vi "Main.vi"(0 "Door open":bool, 5 "Stop":bool, 7 "Start":bool, 9 "Cancel":bool, 11 "Error in":errorcluster) -> (4 "Recipe":i32(listbox), 6 "Cooking":bool, 8 "Power Level":i32, 10 "Buzzer":bool, 14 "Display Panel":string, 15 "Error out":errorcluster)   [LabVIEW 2020, in "Microwave oven.lvlib"]
doc: "This machine is the implementation of microwave oven which will get available food items from a csv file and cook it and display the power level in the front panel indicator"
uses:
  Microwave oven.lvlib
  Typedefs/Queue driver operations.ctl
  Typedefs/Data cluster.ctl
  Typedefs/Number values.ctl
  Typedefs/Timer details.ctl
panel:
  in  "Nine 9":bool
  in  "Eight 8":bool
  in  "Seven 7":bool
  in  "Six 6":bool
  in  "Five 5":bool
  in  "Four 4":bool
  in  "Three 3":bool
  in  "Two 2":bool
  in  "One 1":bool
  # "MICROWAVE OVEN"
  # "MICROWAVE OVEN"
  # "INSTRUCTIONS:\n1. The available recipes are displayed\nin recipes.\n2. You can select the required recipe\nfrom keypad.\n3. Click start to start cooking.\n4. You cannot open the door during\nthe cooking process .\n5. You cannot select another food to \ncook during the cooking process"
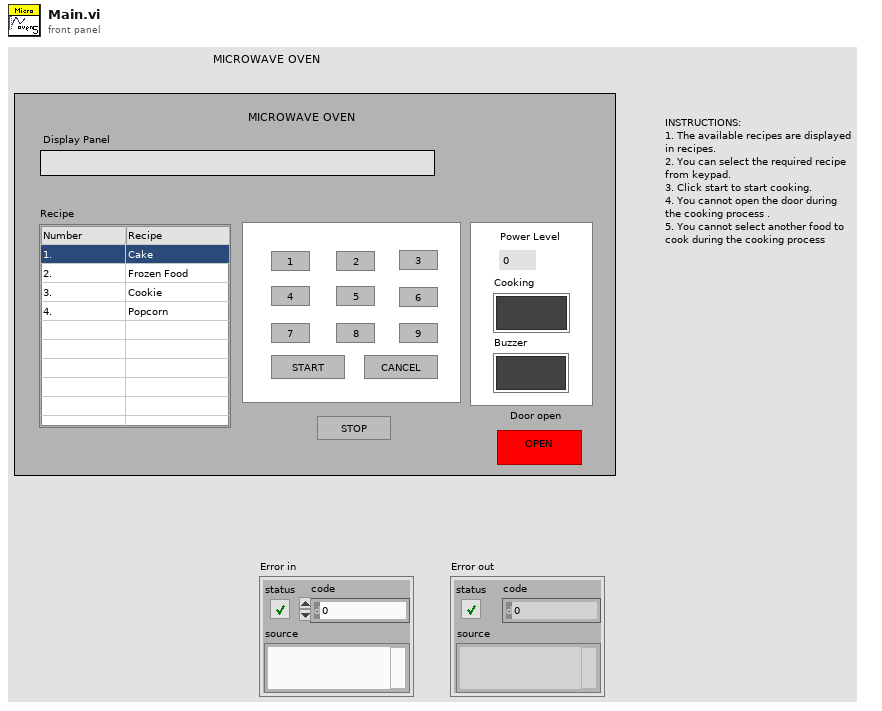
[diagram p1: front panel]
types:
  T1 = typedef "Microwave oven.lvlib/Data cluster.ctl" = cluster{"Number":T2, "Start":bool, "Stop":bool, "Cancel":bool, "Door open":bool, "Power Level":i32, "Display Panel":string, "Cooking":bool, "Buzzer":bool, "Timer details":T3, "Enable controls ref":refnum<vi>[], "Disable controls ref":refnum<vi>[], "Path":path, "Recipe":i32, "Recipie index":i32, "Current Step":i32, "Total Steps":i32, "Recipe Name":string, "Full Recipe":string[], "Recipe Book":string[][], "Cooking time":i32, "Boolean ref":refnum<vi>[]}
  T2 = typedef "Microwave oven.lvlib/Number values.ctl" = cluster{"One":bool, "Two":bool, "Three":bool, "Four":bool, "Five":bool, "Six":bool, "Seven":bool, "Eight":bool, "Nine":bool}
  T3 = typedef "Microwave oven.lvlib/Timer details.ctl" = cluster{"Started?":bool, "Paused":bool, "Start time":dbl, "Set time":dbl, "Previous time":dbl, "Elapsed time":dbl}
  T4 = typedef "Microwave oven.lvlib/Queue driver operations.ctl" = enum16{"Create queue", "Enqueue", "Enstack", "Dequeue", "Flush", "Release"}
  T5 = enum16{"open", "replace", "create", "open or create", "replace or create", "replace or create with confirmation"}
  T6 = enum8{"Enabled", "Disabled", "Disabled and Grayed Out"}
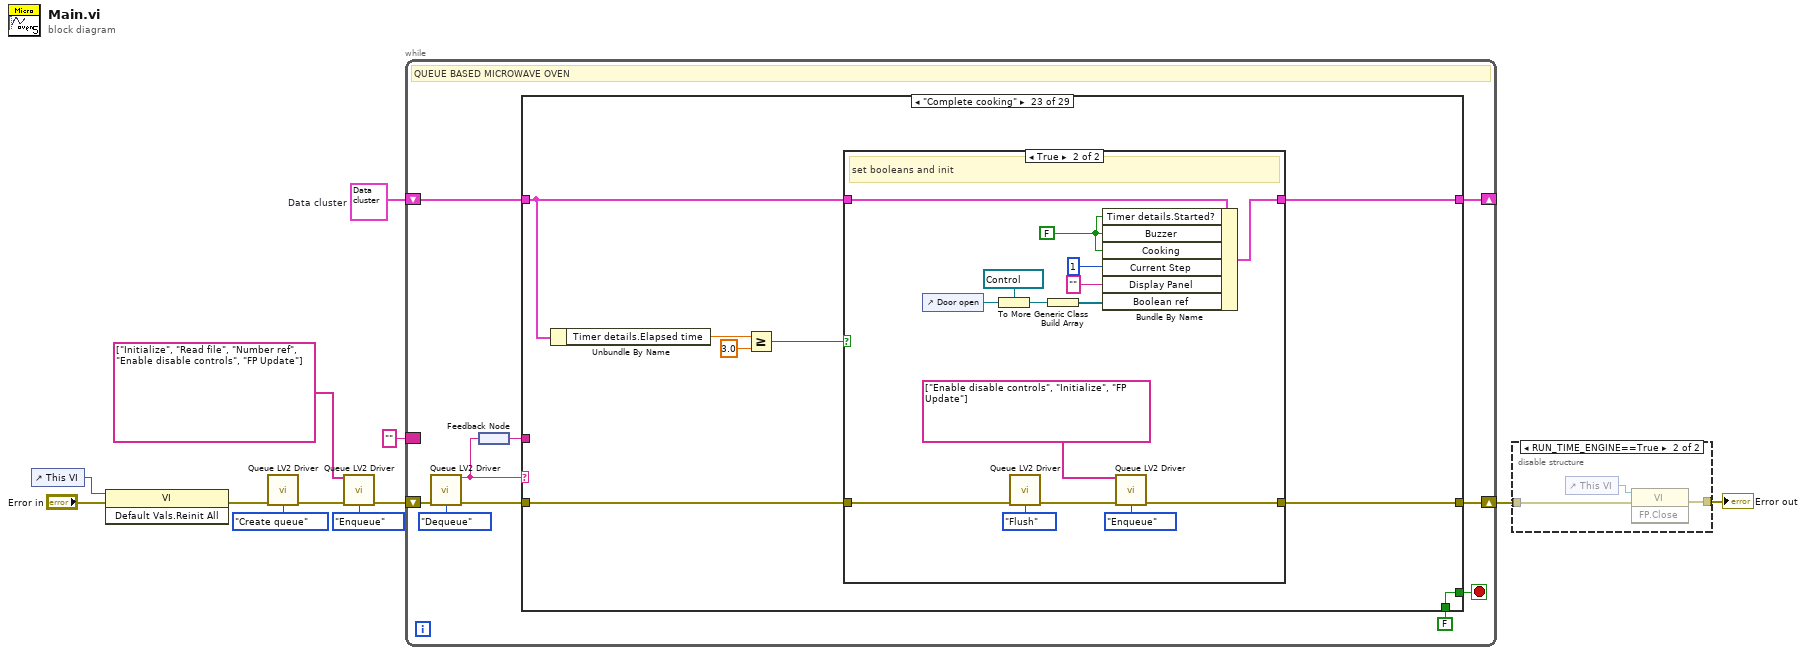
[diagram p0: block diagram]
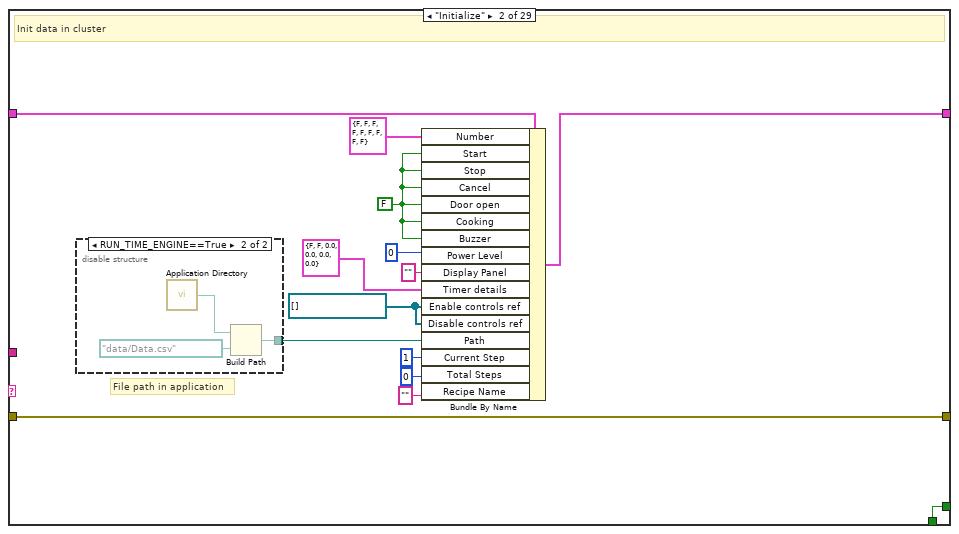
[diagram p4: hidden frame]
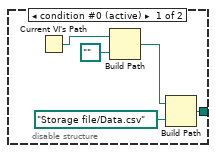
[diagram p5: hidden frame]
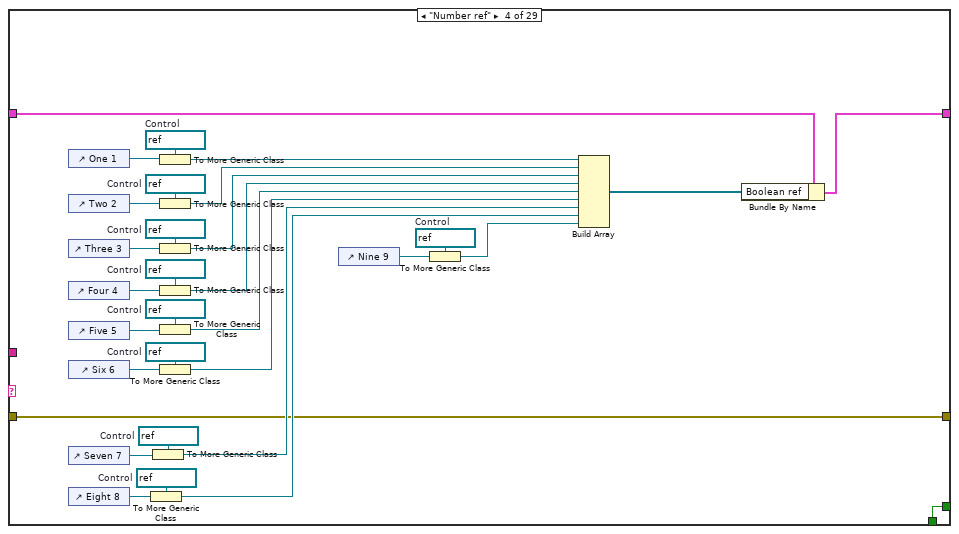
[diagram p7: hidden frame]
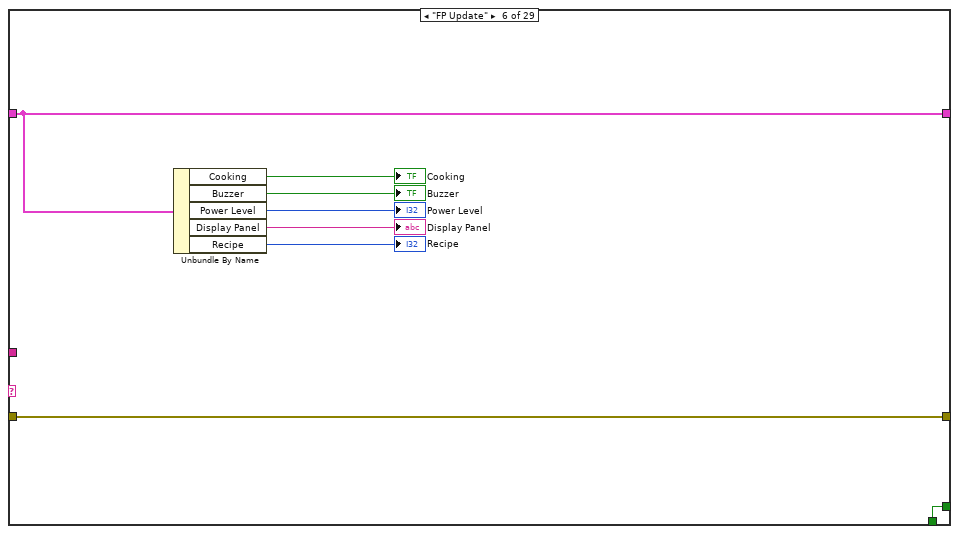
[diagram p9: hidden frame]
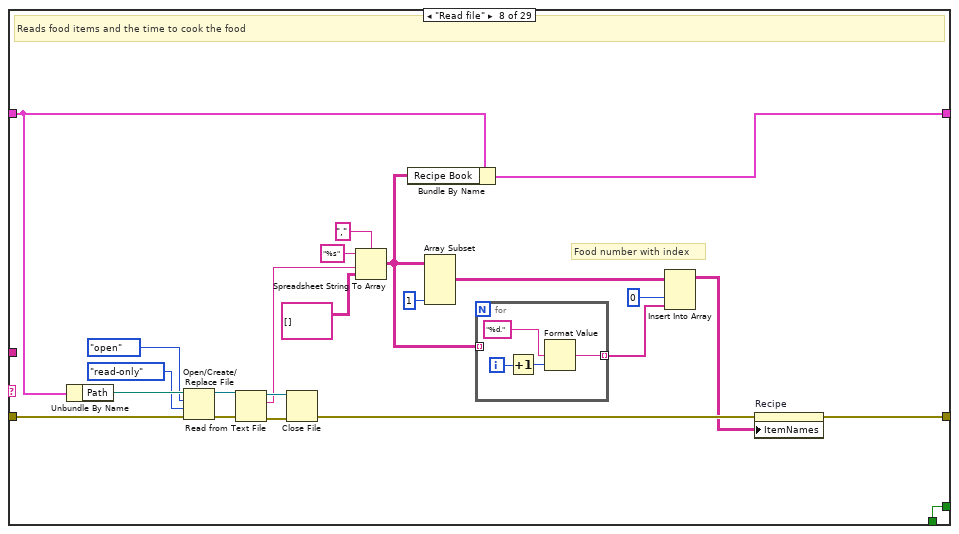
[diagram p11: hidden frame]
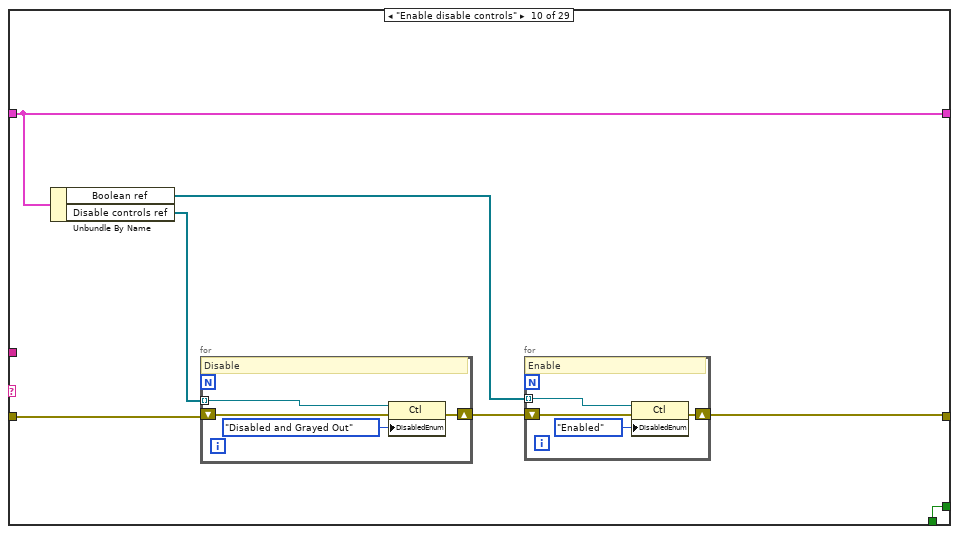
[diagram p13: hidden frame]
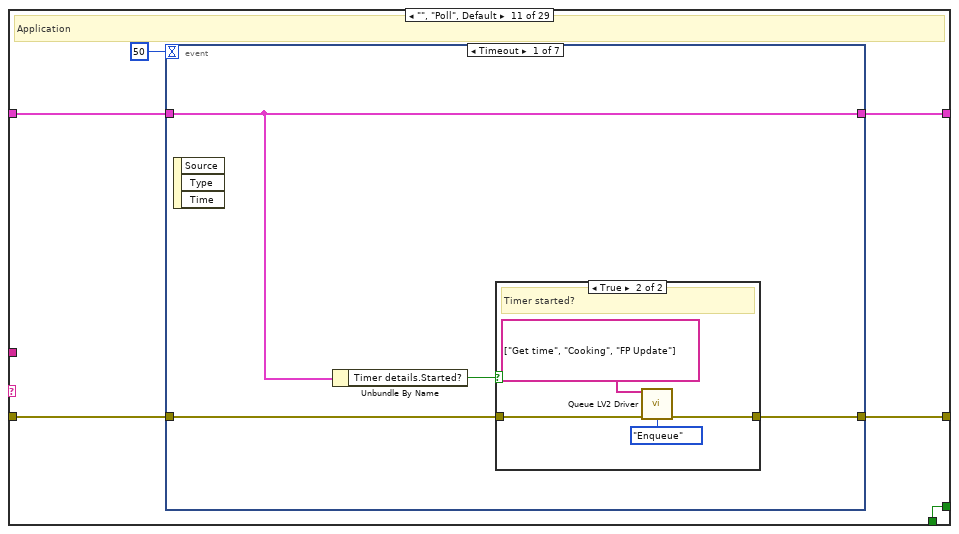
[diagram p14: hidden frame]
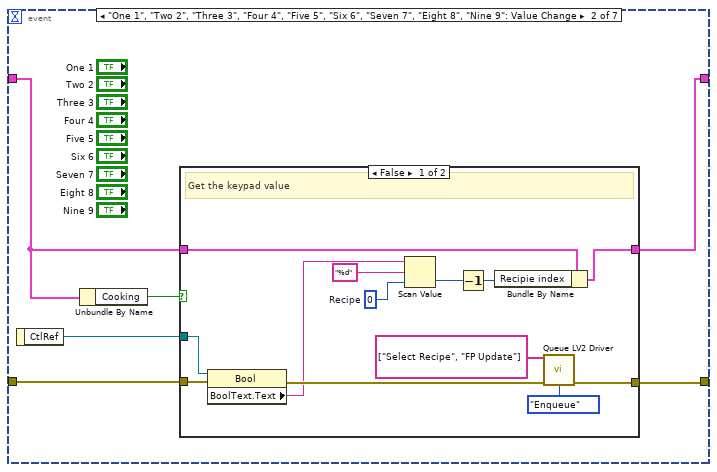
[diagram p16: hidden frame]
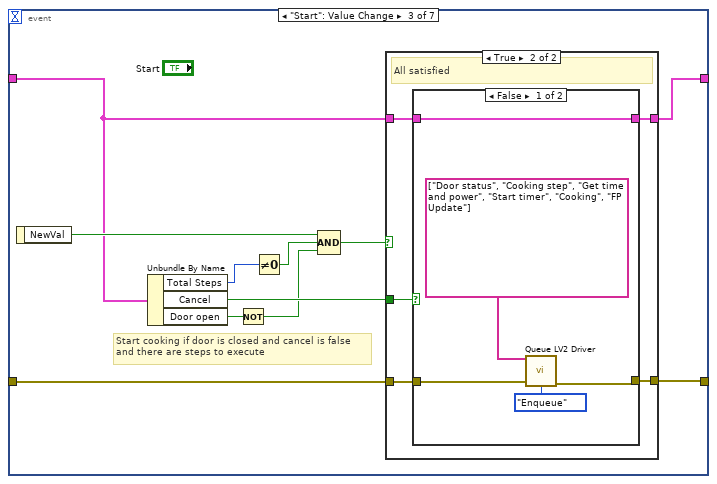
[diagram p18: hidden frame]
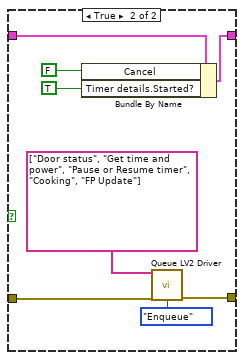
[diagram p20: hidden frame]
diagram:
  w5 = T1 {"Number"={"One"=FALSE, "Two"=FALSE, "Three"=FALSE, "Four"=FALSE, "Five"=FALSE, "Six"=FALSE, "Seven"=FALSE, "Eight"=FALSE, "Nine"=FALSE}, "Start"=FALSE, "Stop"=FALSE, "Cancel"=FALSE, "Door open"=FALSE, "Power Level"=0, "Display Panel"="", "Cooking"=FALSE, "Buzzer"=FALSE, "Timer details"={"Started?"=FALSE, "Paused"=FALSE, "Start time"=0.0, "Set time"=0.0, "Previous time"=0.0, "Elapsed time"=0.0}, "Enable controls ref"=[], "Disable controls ref"=[], "Path"=path "", "Recipe"=0, "Recipie index"=0, "Current Step"=0, "Total Steps"=0, "Recipe Name"="", "Full Recipe"=[], "Recipe Book"=[], "Cooking time"=0, "Boolean ref"=[]}  # Data cluster
  n1 = control-ref of="This VI"() -> (w6:refnum<vi>)
  n2 = invoke class="VI" method="Default Vals.Reinit All"(reference=w6, error in="Error in") -> (error out=w8:errorcluster)  [unwired: 1 in, 2 out]
  n3 = call "Queue LV2 Driver.vi"("Error in"=w8, "Operation"=Queue_driver_operations."Create queue") -> ("Error out"=w10:errorcluster)  [unwired: 12 in, 1 out]
  n4 = call "Queue LV2 Driver.vi"("States"=string[] ["Initialize", "Read file", "Number ref", "Enable disable controls", "FP Update"], "Error in"=w10, "Operation"=Queue_driver_operations."Enqueue") -> ("Error out"=w9:errorcluster)  [unwired: 11 in, 1 out]
  n5 = while {
    shift-right: [w20] -> _
    shift-left: w5 -> [w19]
    border: "" ("Dequeued state") -> [_]
    shift-right: [w18] -> w3
    shift-left: w9 -> [w21]
    stop <- w16 stop-if-true
    # "QUEUE BASED MICROWAVE OVEN"
    n6 = call "Queue LV2 Driver.vi"("Error in"=w21, "Operation"=Queue_driver_operations."Dequeue") -> ("Dequeued state"=w14:string, "Error out"=w17:errorcluster)  [unwired: 12 in]
    n7 = feedback-in #1(w14) -> ()
    n8 = feedback #1() -> (w13:string)
    n9 = case shown="\"Complete cooking\"" w14 {
      tunnel: [w25 w38 w50 w81 w85 w86 w94 w104 w126 w127 w143 w241 w248 w253 w262 w278 w283 w303 w323 w352 w389 w410 w427 w464 w469 w472 w475 w494 w495] -> w20
      tunnel: w19 -> [w25 w39 w50 w82 w85 w86 w94 w105 w126 w127 w142 w241 w249 w254 w264 w278 w281 w304 w326 w353 w388 w411 w428 w464 w469 w472 w475 w494 w495]
      tunnel: [w24 w31 w49 w52 w84 w88 w96 w102 w125 w129 w146 w240 w250 w252 w261 w277 w282 w305 w332 w350 w383 w408 w429 w463 w466 w471 w477 w493 w497] -> w18
      tunnel: w17 -> [w24 w31 w49 w52 w84 w88 w96 w118 w125 w130 w145 w240 w250 w252 w261 w277 w282 w306 w333 w351 w386 w409 w430 w463 w467 w471 w476 w493 w501]
      tunnel: [w23 w33 w48 w51 w83 w87 w95 w119 w124 w128 w147 w239 w251 w255 w268 w276 w287 w310 w337 w355 w390 w413 w434 w462 w465 w470 w480 w492 TRUE] -> w16
      tunnel: FALSE -> [w23 w33 w48 w51 w83 w87 w95 w119 w124 w128 w147 w239 w251 w255 w268 w276 w287 w310 w337 w355 w390 w413 w434 w462 w465 w470 w480 w492 _]
      tunnel: w13 -> [_ _ _ _ _ _ _ _ _ _ _ _ _ _ _ _ _ _ _ _ _ _ _ _ _ _ w481 _ _]
      frame "/***Initialize***/" {
      }
      frame "Initialize" {
        w32 = refnum<vi>[] [] ("Enable controls ref")
        w35 = FALSE ("Door open")
        # "File path in application"
        # "Init data in cluster"
        n10 = disable-structure shown="RUN_TIME_ENGINE==True" {
          disable-tunnel: [w40 w45] -> w26
          frame condition #0 (active) {
            n11 = Current VI's Path() -> (path=w44:path)
            n12 = Build Path(base path=w44, name or relative path=path "..") -> (appended path=w41:path)
            n13 = Build Path(base path=w41, name or relative path=path "Storage file/Data.csv") -> (appended path=w40:path)
          }
          frame condition #1 {
            n14 = call <vilib>:"Application Directory.vi"() -> ("Application Directory"=w46:path)
            n15 = Build Path(base path=w46, name or relative path=path "data/Data.csv") -> (appended path=w45:path)
          }
        }
        n16 = Bundle By Name(cluster=w39, "Number"=T2 {"One"=FALSE, "Two"=FALSE, "Three"=FALSE, "Four"=FALSE, "Five"=FALSE, "Six"=FALSE, "Seven"=FALSE, "Eight"=FALSE, "Nine"=FALSE}, "Start"=w35, "Stop"=w35, "Cancel"=w35, "Door open"=w35, "Cooking"=w35, "Buzzer"=w35, "Power Level"=0, "Display Panel"="", "Timer details"=T3 {"Started?"=FALSE, "Paused"=FALSE, "Start time"=0.0, "Set time"=0.0, "Previous time"=0.0, "Elapsed time"=0.0}, "Enable controls ref"=w32, "Disable controls ref"=w32, "Path"=w26, "Current Step"=1, "Total Steps"=0, "Recipe Name"="") -> (w38:T1)
      }
      frame "/***Getting boolean reference***/" {
      }
      frame "Number ref" {
        w56 = refnum<vi> refnum  # Control
        w67 = refnum<vi> refnum  # Control
        w74 = refnum<vi> refnum  # Control
        w75 = refnum<vi> refnum  # Control
        w76 = refnum<vi> refnum  # Control
        w77 = refnum<vi> refnum  # Control
        w78 = refnum<vi> refnum  # Control
        w79 = refnum<vi> refnum  # Control
        w80 = refnum<vi> refnum  # Control
        n17 = control-ref of="One 1"() -> (w73:refnum<vi>)
        n18 = control-ref of="Two 2"() -> (w72:refnum<vi>)
        n19 = control-ref of="Three 3"() -> (w71:refnum<vi>)
        n20 = control-ref of="Four 4"() -> (w70:refnum<vi>)
        n21 = control-ref of="Five 5"() -> (w69:refnum<vi>)
        n22 = control-ref of="Six 6"() -> (w68:refnum<vi>)
        n23 = control-ref of="Seven 7"() -> (w66:refnum<vi>)
        n24 = control-ref of="Eight 8"() -> (w65:refnum<vi>)
        n25 = To More Generic Class(target class=w67, reference=w65) -> (generic class reference=w57:refnum<vi>)
        n26 = To More Generic Class(target class=w75, reference=w66) -> (generic class reference=w58:refnum<vi>)
        n27 = To More Generic Class(target class=w80, reference=w73) -> (generic class reference=w64:refnum<vi>)
        n28 = To More Generic Class(target class=w79, reference=w72) -> (generic class reference=w63:refnum<vi>)
        n29 = To More Generic Class(target class=w78, reference=w71) -> (generic class reference=w62:refnum<vi>)
        n30 = To More Generic Class(target class=w77, reference=w70) -> (generic class reference=w61:refnum<vi>)
        n31 = To More Generic Class(target class=w76, reference=w69) -> (generic class reference=w60:refnum<vi>)
        n32 = To More Generic Class(target class=w74, reference=w68) -> (generic class reference=w59:refnum<vi>)
        n33 = control-ref of="Nine 9"() -> (w55:refnum<vi>)
        n34 = To More Generic Class(target class=w56, reference=w55) -> (generic class reference=w54:refnum<vi>)
        n35 = Build Array(w64, w63, w62, w61, w60, w59, w58, w57, w54) -> (w53:refnum<vi>[])
        n36 = Bundle By Name(cluster=w82, "Boolean ref"=w53) -> (w81:T1)
      }
      frame "/***FP Related***/" {
      }
      frame "FP Update" {
        n37 = Unbundle By Name(w86) -> ("Cooking"=→"Cooking":bool, "Buzzer"=→"Buzzer":bool, "Power Level"=→"Power Level":i32, "Display Panel"=→"Display Panel":string, "Recipe"=→"Recipe":i32)
      }
      frame "/***Read file***/" {
      }
      frame "Read file" {
        # "Food number with index"
        # "Reads food items and the time to cook the food"
        n38 = Unbundle By Name(w105) -> ("Path"=w117:path)
        n39 = Open/Create/Replace File(file path (use dialog)=w117, error in=w118, operation (0:open)=T5."open", access (0:read/write)=enum16{"read/write", "read-only", "write-only"}."read-only") -> (refnum out=w113:refnum<file>, error out=w114:errorcluster)  [unwired: 2 in, 1 out]
        n40 = Read from Text File(file (use dialog)=w113, error in=w114) -> (refnum out=w111:refnum<file>, text=w107:string, error out=w112:errorcluster)  [unwired: 2 in, 1 out]
        n41 = Close File(refnum=w111, error in=w112) -> (error out=w101:errorcluster)  [unwired: 1 out]
        n42 = Spreadsheet String To Array(delimiter (Tab)=",", format string="%s", spreadsheet string=w107, array type (2D Dbl)=string[][] []) -> (array=w103:string[][])
        n43 = Bundle By Name(cluster=w105, "Recipe Book"=w103) -> (w104:T1)
        n44 = Array Subset(array=w103, length (col)=1 ("length")) -> (w99:string[][])  [unwired: 3 in]
        n45 = for {
          tunnel: w103 -> [_] mode=indexing
          tunnel: [w123] -> w98 mode=indexing
          i -> [w122]
          n46 = Increment(x=w122) -> (x+1=w121:i32)
          n47 = Format Value(format string="%d.", value (0)=w121) -> (output string=w123:string)  [unwired: 1 in]
        }
        n48 = Insert Into Array(array=w99, index (col)=0 ("index (row)"), new element=w98) -> (w97:string[][])  [unwired: 1 in]
        n49 = property on="Recipe" class="MCListbox (strict)"(error in=w101, "ItemNames"=w97) -> (error out=w102:errorcluster)  [unwired: 1 in, 1 out]
      }
      frame "/***Enable and disable controls***/" {
      }
      frame "Enable disable controls" {
        n50 = Unbundle By Name(w127) -> ("Boolean ref"=w132:refnum<vi>[], "Disable controls ref"=w131:refnum<vi>[])
        n51 = for {
          shift-right: [w140] -> w133
          shift-left: w130 -> [w141]
          tunnel: w131 -> [w139] mode=indexing
          # "Disable"
          n52 = property class="Ctl"(reference=w139, error in=w141, "DisabledEnum"=T6."Disabled and Grayed Out" ("Disabled")) -> (error out=w140:errorcluster)  [unwired: 1 out]
        }
        n53 = for {
          shift-right: [w136] -> w129
          shift-left: w133 -> [w137]
          tunnel: w132 -> [w135] mode=indexing
          # "Enable"
          n54 = property class="Ctl"(reference=w135, error in=w137, "DisabledEnum"=T6."Enabled" ("Disabled")) -> (error out=w136:errorcluster)  [unwired: 1 out]
        }
      }
      frame "", "Poll", Default {
        # "Application"
        n55 = event shown="[0] Timeout" {
          selector: _ -> [_ _ _ _ _ _ _]
          dyn-events: _ -> [_ _ _ _ _ _ _]
          timeout: 50 -> [_ _ _ _ _ _ _]
          tunnel: [w150 w160 w181 w210 w225 w229 w234] -> w146
          tunnel: w145 -> [w151 w162 w180 w211 w225 w230 w235]
          tunnel: [w149 w159 w183 w212 w224 w232 w233] -> w143
          tunnel: w142 -> [w149 w158 w184 w213 w227 w232 w233]
          event Timeout {
            n56 = event-data() -> ()  [unwired: 1 in, 3 out]
            n57 = Unbundle By Name(w149) -> ("Timer details.Started?"=w148:bool)
            n58 = case shown="True" w148 {
              tunnel: w151 -> [w152 w155]
              tunnel: [w152 w154] -> w150
              frame False {
                # "Not started"
              }
              frame True {
                # "Timer started?"
                n59 = call "Queue LV2 Driver.vi"("States"=string[] ["Get time", "Cooking", "FP Update"], "Error in"=w155, "Operation"=Queue_driver_operations."Enqueue") -> ("Error out"=w154:errorcluster)  [unwired: 11 in, 1 out]
              }
            }
          }
          event "One 1", "Two 2", "Three 3", "Four 4", "Five 5", "Six 6", "Seven 7", "Eight 8", "Nine 9": Value Change {
            n60 = event-data() -> ("CtlRef"=w161:refnum<vi>)  [unwired: 1 in]
            n61 = Unbundle By Name(w158) -> ("Cooking"=w157:bool)
            n62 = case shown="False" w157 {
              tunnel: w162 -> [w175 w176]
              tunnel: w161 -> [w174 _]
              tunnel: [w172 w176] -> w160
              tunnel: w158 -> [w164 w177]
              tunnel: [w163 w177] -> w159
              frame False {
                w168 = 0  # Recipe
                # "Get the keypad value"
                n63 = property class="Bool"(reference=w174, error in=w175) -> (error out=w173:errorcluster, "BoolText.Text"=w166:string)  [unwired: 1 out]
                n64 = Scan Value(string=w166, format string="%d", default (0 dbl)=w168) -> (value=w167:i32)  [unwired: 1 out]
                n65 = Decrement(x=w167) -> (x-1=w165:i32)
                n66 = Bundle By Name(cluster=w164, "Recipie index"=w165) -> (w163:T1)
                n67 = call "Queue LV2 Driver.vi"("States"=string[] ["Select Recipe", "FP Update"], "Error in"=w173, "Operation"=Queue_driver_operations."Enqueue") -> ("Error out"=w172:errorcluster)  [unwired: 11 in, 1 out]
              }
              frame True {
                # "If cooking is in progess"
              }
            }
          }
          event "Start": Value Change {
            # "Start cooking if door is closed and cancel is false\nand there are steps to execute"
            n68 = event-data() -> ("NewVal"=w187:bool)  [unwired: 1 in]
            n69 = Unbundle By Name(w184) -> ("Total Steps"=w186:i32, "Cancel"=w182:bool, "Door open"=w179:bool)
            n70 = Not(x=w179) -> (.not. x?=w178:bool)
            n71 = Not Equal To 0?(x=w186) -> (x != 0?=w185:bool)
            n72 = Compound Arithmetic op=AND(w187, w185, w178) -> (w188:bool)
            n73 = case shown="True" w188 {
              tunnel: w184 -> [w190 w192]
              tunnel: [w190 w191] -> w183
              tunnel: w182 -> [_ w195]
              tunnel: [w189 w194] -> w181
              tunnel: w180 -> [w189 w193]
              frame False {
                # "If any of the one fails"
              }
              frame True {
                # "All satisfied"
                n74 = case shown="False" w195 {
                  tunnel: [w197 w207] -> w194
                  tunnel: w193 -> [w198 w206]
                  tunnel: w192 -> [w200 w205]
                  tunnel: [w200 w204] -> w191
                  frame False {
                    n75 = call "Queue LV2 Driver.vi"("States"=string[] ["Door status", "Cooking step", "Get time and power", "Start timer", "Cooking", "FP Update"], "Error in"=w198, "Operation"=Queue_driver_operations."Enqueue") -> ("Error out"=w197:errorcluster)  [unwired: 11 in, 1 out]
                  }
                  frame True {
                    n76 = Bundle By Name(cluster=w205, "Cancel"=FALSE, "Timer details.Started?"=TRUE) -> (w204:T1)
                    n77 = call "Queue LV2 Driver.vi"("States"=string[] ["Door status", "Get time and power", "Pause or Resume timer", "Cooking", "FP Update"], "Error in"=w206, "Operation"=Queue_driver_operations."Enqueue") -> ("Error out"=w207:errorcluster)  [unwired: 11 in, 1 out]
                  }
                }
              }
            }
          }
          event "Cancel": Value Change {
            n78 = event-data() -> ("NewVal"=w209:bool)  [unwired: 1 in]
            n79 = case shown="False" w209 {
              tunnel: w213 -> [w214 w223]
              tunnel: [w214 w222] -> w212
              tunnel: w211 -> [w215 w218]
              tunnel: [w215 w217] -> w210
              frame False {
              }
              frame True {
                # "Pause cooking"
                n80 = Bundle By Name(cluster=w223, "Cancel"=TRUE, "Timer details.Started?"=FALSE) -> (w222:T1)
                n81 = call "Queue LV2 Driver.vi"("States"=string[] ["Pause or Resume timer", "Pause cooking"], "Error in"=w218, "Operation"=Queue_driver_operations."Enqueue") -> ("Error out"=w217:errorcluster)  [unwired: 11 in, 1 out]
              }
            }
          }
          event "Door open": Value Change {
            n82 = event-data() -> ("NewVal"=w226:bool)  [unwired: 1 in]
            n83 = Bundle By Name(cluster=w227, "Door open"=w226) -> (w224:T1)
          }
          event "Stop": Value Change {
            n84 = event-data() -> ()  [unwired: 1 in, 1 out]
            n85 = call "Queue LV2 Driver.vi"("States"=string[] ["Reinit", "Exit"], "Error in"=w230, "Operation"=Queue_driver_operations."Enqueue") -> ("Error out"=w229:errorcluster)  [unwired: 11 in, 1 out]
          }
          event Panel Close? {
            n86 = event-data() -> ()  [unwired: 1 in, 1 out]
            n87 = call "Queue LV2 Driver.vi"("States"=string[] ["Reinit", "Exit"], "Error in"=w235, "Operation"=Queue_driver_operations."Enqueue") -> ("Error out"=w234:errorcluster)  [unwired: 11 in, 1 out]
            n88 = event-data("Discard?"=TRUE) -> ()  [unwired: 1 in, 1 out]
          }
        }
      }
      frame "/***Timing states***/" {
      }
      frame "Start timer" {
        w245 = 0.0 ("Timer details.Previous time")
        n89 = Unbundle By Name(w249) -> ("Timer details.Started?"=w243:bool)
        n90 = Not(x=w243) -> (.not. x?=w242:bool)
        n91 = Get Date/Time In Seconds() -> (seconds since 1Jan1904=w246:timestamp)
        n92 = To Double Precision Float(number=w246) -> (double precision float=w247:dbl)
        n93 = Bundle By Name(cluster=w249, "Timer details.Start time"=w247, "Timer details.Set time"=w245, "Timer details.Previous time"=w245, "Timer details.Started?"=w242, "Timer details.Paused"=FALSE) -> (w248:T1)
      }
      frame "Pause or Resume timer" {
        n94 = in-place {
          n95 = in-place-cluster #2(w254) -> ("Timer details.Paused"=w258:bool, "Timer details.Elapsed time"=w256:dbl)  [unwired: 2 out]
          n96 = Get Date/Time In Seconds() -> (seconds since 1Jan1904=w260:timestamp)
          n97 = Not(x=w258) -> (.not. x?=w257:bool)
          n98 = To Double Precision Float(number=w260) -> (double precision float=w259:dbl)
          n99 = in-place-cluster #2("Timer details.Start time"=w259, "Timer details.Paused"=w257, "Timer details.Elapsed time"=w256, "Timer details.Previous time"=w256) -> (w253:T1)
        }
      }
      frame "Get time" {
        n100 = Unbundle By Name(w264) -> ("Timer details.Paused"=w266:bool, "Timer details.Start time"=w267:dbl, "Timer details.Previous time"=w265:dbl)
        n101 = case "Paused?" shown="False" w266 {
          tunnel: [w273 w275] -> w263
          tunnel: w267 -> [w270 _]
          tunnel: w265 -> [w269 w275]
          frame False {
            # "Get the elapsed time"
            n102 = Get Date/Time In Seconds() -> (seconds since 1Jan1904=w271:timestamp)
            n103 = To Double Precision Float(number=w271) -> (double precision float=w272:dbl)
            n104 = Subtract(x=w272, y=w270) -> (x-y=w274:dbl)
            n105 = Add(x=w274, y=w269) -> (x+y=w273:dbl)
          }
          frame True {
            # "Give same value if timer paused"
          }
        }
        n106 = Bundle By Name(cluster=w264, "Timer details.Elapsed time"=w263) -> (w262:T1)
      }
      frame "/***Cooking states***/" {
      }
      frame "Select Recipe" {
        # "Keypad input to select recipe and update in FP"
        n107 = Unbundle By Name(w281) -> ("Recipe Book"=w286:string[][], "Recipie index"=w285:i32)
        n108 = Index Array(array=w286, index (row)=w285) -> (element=w279:string[])  [unwired: 1 in]
        n109 = Bundle By Name(cluster=w281, "Full Recipe"=w279) -> (w280:T1)
        n110 = Empty Array?(array=w279) -> (empty?=w284:bool)
        n111 = case shown="False" w284 {
          tunnel: w279 -> [w293 _]
          tunnel: w280 -> [w291 w302]
          tunnel: [w288 w300] -> w283
          frame False {
            # "Valid food"
            n112 = for {
              tunnel: w293 -> [w296] mode=indexing
              tunnel: [w295] -> w290
              i -> [w297]
              stop <- w294 stop-if-true
              n113 = Empty String/Path?(string/path=w296) -> (empty?=w294:bool)
              n114 = Decrement(x=w297) -> (x-1=w298:i32)
              n115 = Select(t=w298, s=w294, f=w297) -> (s? t:f=w295:i32)
            }
            n116 = Index Array(array=w293, index=0) -> (element=w289:string)
            n117 = Bundle By Name(cluster=w291, "Recipe Name"=w289, "Display Panel"=w289, "Total Steps"=w290) -> (w288:T1)
          }
          frame True {
            # "If there is no food"
            n118 = Bundle By Name(cluster=w302, "Display Panel"="No Recipe", "Total Steps"=0) -> (w300:T1)
          }
        }
      }
      frame "Cooking step" {
        # "Check if there are still steps to continue cooking"
        n119 = Unbundle By Name(w304) -> ("Current Step"=w309:i32, "Total Steps"=w308:i32)
        n120 = Greater?(x=w309, y=w308) -> (0:w307:bool)
        n121 = case shown="True" w307 {
          tunnel: w306 -> [w311 w320]
          tunnel: [w311 w318] -> w305
          tunnel: w304 -> [w312 w316]
          tunnel: [w312 w314] -> w303
          frame False {
            # "Continue"
          }
          frame True {
            w313 = FALSE ("Cooking")
            # "If there is no cooking step then complete cooking"
            n122 = Bundle By Name(cluster=w316, "Buzzer"=TRUE, "Cooking"=w313, "Timer details.Started?"=w313) -> (w314:T1)
            n123 = call "Queue LV2 Driver.vi"("Error in"=w320, "Operation"=Queue_driver_operations."Flush") -> ("Error out"=w319:errorcluster)  [unwired: 12 in, 1 out]
            n124 = call "Queue LV2 Driver.vi"("States"=string[] ["Start timer", "Complete cooking", "FP Update"] ("States s[]"), "Error in"=w319, "Operation"=Queue_driver_operations."Enqueue") -> ("Error out"=w318:errorcluster)  [unwired: 11 in, 1 out]
          }
        }
      }
      frame "Get time and power" {
        # "Extract time"
        # "Calculate time from csv"
        n125 = Unbundle By Name(w326) -> ("Full Recipe"=w336:string[], "Current Step"=w335:i32)
        n126 = Index Array(array=w336, index=w335) -> (element=w334:string)
        n127 = Scan From String(format string="%dPL%d", input string=w334, error in=w333) -> (error out=w332:errorcluster, output 1=w330:i32, output 2=w325:i32)  [unwired: 3 in, 2 out]
        n128 = Quotient & Remainder(x=w330, y=100) -> (x-y*floor(x/y)=w328:i32, floor(x/y)=w327:i32)
        n129 = case shown="0..59, Default" w328 {
          selector: w328 -> [w339 w345]
          tunnel: w327 -> [w340 w344]
          tunnel: [w338 w343] -> w324
          frame 0..59, Default {
            # "values less than 60"
            n130 = Multiply(x=w340, y=60) -> (x*y=w342:i32)
            n131 = Add(x=w339, y=w342) -> (x+y=w338:i32)
          }
          frame 60.. {
            w346 = 60 ("y")
            # "values greater than 60"
            n132 = Increment(x=w344) -> (x+1=w348:i32)
            n133 = Subtract(x=w345, y=w346) -> (x-y=w349:i32)
            n134 = Multiply(x=w348, y=w346) -> (x*y=w347:i32)
            n135 = Add(x=w349, y=w347) -> (x+y=w343:i32)
          }
        }
        n136 = Bundle By Name(cluster=w326, "Cooking time"=w324, "Power Level"=w325) -> (w323:T1)
      }
      frame "Door status" {
        n137 = Unbundle By Name(w353) -> ("Door open"=w354:bool)
        n138 = case shown="True" w354 {
          tunnel: w353 -> [w365 w366]
          tunnel: [w364 w366] -> w352
          tunnel: w351 -> [w358 w368]
          tunnel: [w357 w367] -> w350
          frame False {
            # "If door closed disable it"
            n139 = control-ref of="Door open"() -> (w360:refnum<vi>)
            n140 = To More Generic Class(target class=refnum<vi> refnum ("reference"), reference=w360) -> (generic class reference=w362:refnum<vi>)
            n141 = call "Queue LV2 Driver.vi"("States"=string[] ["Enable disable controls"], "Error in"=w358, "Operation"=Queue_driver_operations."Enqueue") -> ("Error out"=w357:errorcluster)  [unwired: 11 in, 1 out]
            n142 = Build Array(w362) -> (w363:refnum<vi>[])
            n143 = Bundle By Name(cluster=w365, "Disable controls ref"=w363) -> (w364:T1)
          }
          frame True {
            # "If door is open pause cooking"
            n144 = call "Queue LV2 Driver.vi"("Error in"=w368, "Operation"=Queue_driver_operations."Flush") -> ("Error out"=w367:errorcluster)  [unwired: 12 in, 1 out]
          }
        }
      }
      frame "Cooking" {
        # "Cooking process"
        n145 = Unbundle By Name(w388) -> ("Current Step"=w379:i32, "Timer details.Elapsed time"=w370:dbl, "Cooking time"=w381:i32, "Recipe Name"=w385:string, "Total Steps"=w378:i32, "Cooking time"=w371:i32)
        n146 = To Double Precision Float(number=w371) -> (double precision float=w374:dbl)
        n147 = Subtract(x=w374, y=w370) -> (x-y=w373:dbl)
        n148 = To Double Precision Float(number=w381) -> (double precision float=w382:dbl)
        n149 = Format Date/Time String(time format string (%c)="%M : %S", seconds (now)=w373, UTC format=TRUE) -> (date/time string=w372:string)
        n150 = Format Into String(format string=" Step %d of %d Time %s", initial string=w385, error in=w386, w379, w378, w372) -> (resulting string=w377:string, error out=w384:errorcluster)
        n151 = Greater?(x=w370, y=w382) -> (0:w380:bool)
        n152 = case shown="True" w380 {
          tunnel: [w397 w406] -> w389
          tunnel: w388 -> [w398 w407]
          tunnel: w384 -> [w395 w401]
          tunnel: [w394 w400] -> w383
          tunnel: w379 -> [_ w405]
          tunnel: w377 -> [w391 _]
          frame False {
            # "continue if cooking is not completed"
            n153 = Bundle By Name(cluster=w398, "Display Panel"=w391, "Cooking"=TRUE) -> (w397:T1)
            n154 = call "Queue LV2 Driver.vi"("States"=string[] ["FP Update", "Get time"], "Error in"=w395, "Operation"=Queue_driver_operations."Enqueue") -> ("Error out"=w394:errorcluster)  [unwired: 11 in, 1 out]
          }
          frame True {
            w403 = 0.0 ("Timer details.Elapsed time")
            # "go to next step if cooking time completes"
            n155 = Increment(x=w405) -> (x+1=w404:i32)
            n156 = Bundle By Name(cluster=w407, "Current Step"=w404, "Timer details.Elapsed time"=w403, "Timer details.Previous time"=w403) -> (w406:T1)
            n157 = call "Queue LV2 Driver.vi"("States"=string[] ["Cooking step", "Get time and power", "Start timer", "FP Update"], "Error in"=w401, "Operation"=Queue_driver_operations."Enqueue") -> ("Error out"=w400:errorcluster)  [unwired: 11 in, 1 out]
          }
        }
      }
      frame "Pause cooking" {
        n158 = Unbundle By Name(w411) -> ("Cancel"=w412:bool)
        n159 = case shown="True" w412 {
          tunnel: w411 -> [w414 w426]
          tunnel: [w414 w423] -> w410
          tunnel: w409 -> [w417 w421]
          tunnel: [w416 w420] -> w408
          frame False {
            # "Else continue"
            n160 = call "Queue LV2 Driver.vi"("States"=string[] ["FP Update", "Get time and power"], "Error in"=w417, "Operation"=Queue_driver_operations."Enqueue") -> ("Error out"=w416:errorcluster)  [unwired: 11 in, 1 out]
          }
          frame True {
            # "Pause if cancel is pressed"
            n161 = call "Queue LV2 Driver.vi"("States"=string[] ["FP Update"], "Error in"=w421, "Operation"=Queue_driver_operations."Enqueue") -> ("Error out"=w420:errorcluster)  [unwired: 11 in, 1 out]
            n162 = Bundle By Name(cluster=w426, "Cooking"=FALSE, "Power Level"=0) -> (w423:T1)
          }
        }
      }
      frame "Complete cooking" {
        n163 = Unbundle By Name(w428) -> ("Timer details.Elapsed time"=w433:dbl)
        n164 = Greater Or Equal?(x=w433, y=3.0) -> (x >= y?=w431:bool)
        n165 = case shown="True" w431 {
          tunnel: w430 -> [w445 w456]
          tunnel: [w444 w452] -> w429
          tunnel: w428 -> [w443 w461]
          tunnel: [w442 w458] -> w427
          frame False {
            # "wait until elapsed time reaches 3"
            n166 = Bundle By Name(cluster=w443, "Power Level"=0, "Buzzer"=TRUE, "Cooking"=FALSE, "Display Panel"="Done !", "Timer details.Elapsed time"=1.0, "Timer details.Paused"=FALSE) -> (w442:T1)
            n167 = call "Queue LV2 Driver.vi"("States"=string[] ["FP Update", "Get time", "Complete cooking"], "Error in"=w445, "Operation"=Queue_driver_operations."Enqueue") -> ("Error out"=w444:errorcluster)  [unwired: 11 in, 1 out]
          }
          frame True {
            w451 = FALSE ("Buzzer")
            # "set booleans and init"
            n168 = control-ref of="Door open"() -> (w447:refnum<vi>)
            n169 = To More Generic Class(target class=refnum<vi> refnum ("reference"), reference=w447) -> (generic class reference=w450:refnum<vi>)
            n170 = call "Queue LV2 Driver.vi"("Error in"=w456, "Operation"=Queue_driver_operations."Flush") -> ("Error out"=w454:errorcluster)  [unwired: 12 in, 1 out]
            n171 = Build Array(w450) -> (w448:refnum<vi>[])
            n172 = Bundle By Name(cluster=w461, "Timer details.Started?"=w451, "Buzzer"=w451, "Cooking"=w451, "Current Step"=1, "Display Panel"="", "Boolean ref"=w448) -> (w458:T1)
            n173 = call "Queue LV2 Driver.vi"("States"=string[] ["Enable disable controls", "Initialize", "FP Update"], "Error in"=w454, "Operation"=Queue_driver_operations."Enqueue") -> ("Error out"=w452:errorcluster)  [unwired: 11 in, 1 out]
          }
        }
      }
      frame "/*** Reinit values upon exit" {
      }
      frame "Reinit" {
        # "Reinit values during exit"
        n174 = control-ref of="This VI"() -> (w468:refnum<vi>)
        n175 = invoke class="VI" method="Default Vals.Reinit All"(reference=w468, error in=w467) -> (error out=w466:errorcluster)  [unwired: 1 in, 2 out]
      }
      frame "/***Error***/" {
      }
      frame "Error" {
        # "Handle error"
        n176 = Unbundle By Name(w476) -> ("code"=w484:i32, "source"=w483:string)
        n177 = call <vilib>:"Clear Errors.vi"("error in (no error)"=w476, "specific error code to clear (0: all)"=w484) -> ("error out"=w486:errorcluster)  [unwired: 4 in, 1 out]
        n178 = Format Into String(format string="Error occurred in state \"%s\"!!\nError Code: %d\nError Source: %s\n\nDo you wish to continue?", error in=w486, w481, w484, w483) -> (resulting string=w482:string, error out=w478:errorcluster)  [unwired: 1 in]
        n179 = Two Button Dialog(message=w482, 1:"Exit" ("F button name (\"Cancel\")"), 2:"Continue" ("T button name (\"OK\")")) -> (T button?=w479:bool)
        n180 = case shown="False" w479 {
          tunnel: w478 -> [w490 w491]
          tunnel: [w489 w491] -> w477
          frame False {
            # "Exit"
            n181 = call "Queue LV2 Driver.vi"("States"=string[] ["Reinit", "Exit"], "Error in"=w490, "Operation"=Queue_driver_operations."Enqueue") -> ("Error out"=w489:errorcluster)  [unwired: 11 in, 1 out]
          }
          frame True {
            # "Continue"
          }
        }
      }
      frame "/***Exit***/" {
      }
      frame "Exit" {
        # "Flush and release queue"
        # "Exit"
        n182 = call "Queue LV2 Driver.vi"("Error in"=w501, "Operation"=Queue_driver_operations."Flush") -> ("Error out"=w500:errorcluster)  [unwired: 12 in, 1 out]
        n183 = call "Queue LV2 Driver.vi"("Error in"=w500, "Operation"=Queue_driver_operations."Release") -> ("Error out"=w497:errorcluster)  [unwired: 12 in, 1 out]
      }
    }
  }
  n184 = disable-structure shown="RUN_TIME_ENGINE==True" {
    disable-tunnel: w3 -> [w502 w505]
    disable-tunnel: [w502 w504] -> w2
    frame condition #0 (active) {
    }
    frame condition #1 {
      n185 = control-ref of="This VI"() -> (w503:refnum<vi>)
      n186 = invoke class="VI" method="FP.Close"(reference=w503, error in=w505) -> (error out=w504:errorcluster)  [unwired: 1 in, 2 out]
    }
  }
  "Error out" <- w2
